vi "Update test_serialize_deserialize Poly Selector.vi"(8 "error in (no error)":errorcluster, 11 "Diagram in":refnum<vi>) -> (0 "error out":errorcluster, 3 "Diagram out":refnum<vi>)   [LabVIEW 2020]
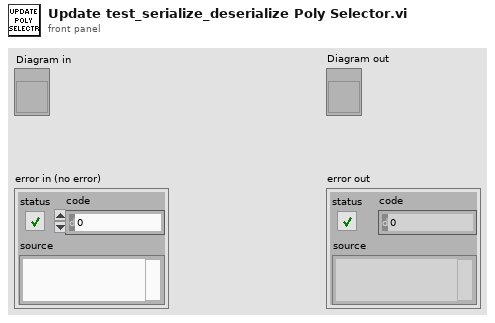
[diagram p1: front panel]
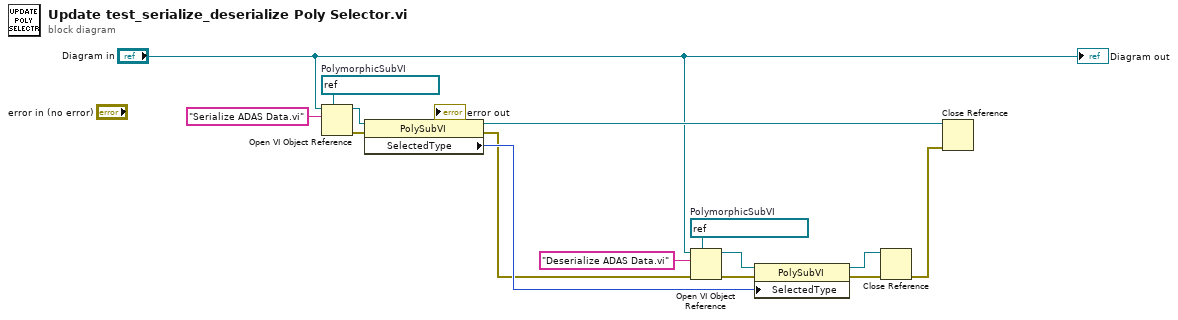
[diagram p0: block diagram]
diagram:
  w6 = refnum<vi> refnum  # PolymorphicSubVI
  w3 = refnum<vi> refnum  # PolymorphicSubVI
  n1 = Open VI Object Reference(7:w3, 10:"Serialize ADAS Data.vi" ("name/order"), 11:"Diagram in") -> (0:w10:errorcluster, 3:w4:refnum<vi>)  [unwired: 1 in]
  n2 = property class="PolySubVI"(reference=w4, error in=w10) -> (reference out=w14:refnum<vi>, error out=w1:errorcluster, "SelectedType"=w9:i32)
  n3 = Open VI Object Reference(7:w6, 8:w1, 10:"Deserialize ADAS Data.vi" ("name/order"), 11:"Diagram in") -> (0:w11:errorcluster, 3:w8:refnum<vi>)
  n4 = property class="PolySubVI"(reference=w8, error in=w11, "SelectedType"=w9) -> (reference out=w15:refnum<vi>, error out=w12:errorcluster)
  n5 = Close Reference(reference=w15, error in (no error)=w12) -> (error out=w13:errorcluster)
  n6 = Close Reference(reference=w14, error in (no error)=w13) -> ()  [unwired: 1 out]
  "Diagram out" <- "Diagram in"
